vi "SDG60ConfBurstSplit.vi"() -> ()   [LabVIEW 2018]
panel:
  in  "Gate Polarity 0: Positive":u16(ring) items=["Positive", "Negative"]
  in  "Burst Delay (1.352 us)":dbl=1.352e-06
  in  "Triggered/Gated: (0:Triggered)":i32(ring) items=["Triggered", "Gated"]
  in  "Trigger Out Mode (0: Off)":u16(ring) items=["Off", "Rise", "Fall"]
  in  "Trigger Source (0: Internal)":i32(ring) items=["Internal", "External", "Manual"]
  in  "Start Phase (0.0 degrees)":dbl min=0.0 max=360.0 format="%#.15g"
  in  "Channel (1:Channel 1)":i32(ring)=1 items=["Channel 1"=1, "Channel 2"=2]
  in  "Enable Burst (T: Enable)":bool=TRUE
  in  "error in (no error)":errorcluster
  out "error out":errorcluster
  in  "VISA resource name":refnum<visa-resource-name>="USB0::0xF4EC::0x1101::SDG6XEBC5R0119::INSTR"
  out "VISA resource name out":refnum<visa-resource-name>
  # "Trigger out ignored when gated \nand/or TrigSrc is Ext"
  # "Res: 0.1degrees"
  # "Range: 1.352us-100s\nLimited by frequency\n6 digits precision"
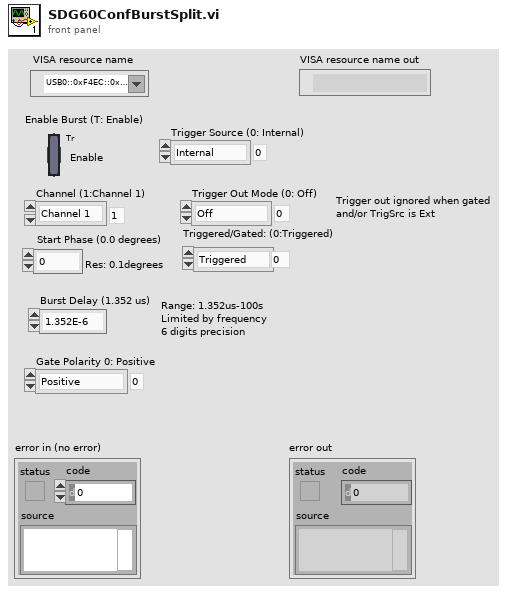
[diagram p1: front panel]
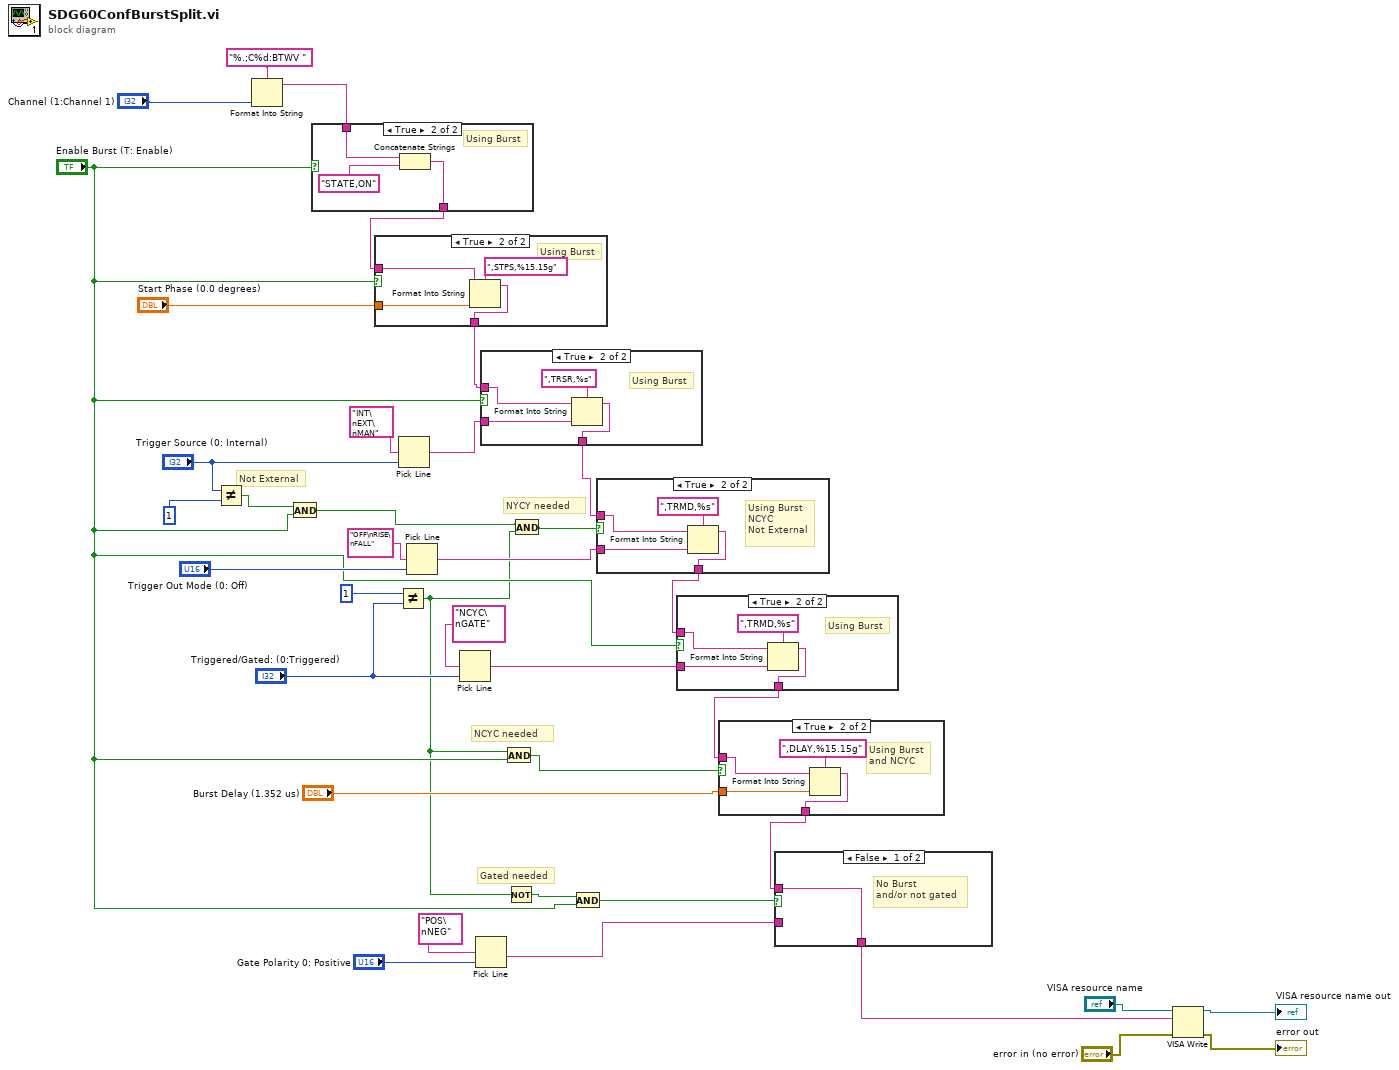
[diagram p0: block diagram]
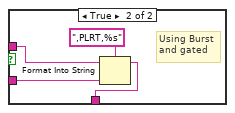
[diagram p2: hidden frame]
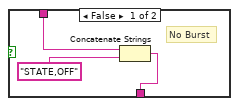
[diagram p8: hidden frame]
diagram:
  # "Gated needed"
  # "NCYC needed"
  # "NYCY needed"
  # "Not External"
  n1 = Not Equal?(x="Trigger Source (0: Internal)", y=1) -> (x != y?=w13:bool)
  n2 = Format Into String(format string="%.;C%d:BTWV ", "Channel (1:Channel 1)") -> (resulting string=w36:string)  [unwired: 2 in, 1 out]
  n3 = And(x=w13, y="Enable Burst (T: Enable)") -> (x .and. y?=w11:bool)
  n4 = case shown="True" "Enable Burst (T: Enable)" {
    tunnel: w36 -> [w41 w44]
    tunnel: [w39 w42] -> w35
    frame False {
      # "No Burst"
      n5 = Concatenate Strings(w41, "STATE,OFF") -> (w39:string)
    }
    frame True {
      # "Using Burst"
      n6 = Concatenate Strings(w44, "STATE,ON") -> (w42:string)
    }
  }
  n7 = case shown="True" "Enable Burst (T: Enable)" {
    tunnel: w35 -> [w45 w48]
    tunnel: [w45 w46] -> w30
    tunnel: "Start Phase (0.0 degrees)" -> [_ w49]
    frame False {
      # "No Burst"
    }
    frame True {
      # "Using Burst"
      n8 = Format Into String(format string=",STPS,%15.15g", initial string=w48, w49) -> (resulting string=w46:string)  [unwired: 1 in, 1 out]
    }
  }
  n9 = Not Equal?(x=1, y="Triggered/Gated: (0:Triggered)") -> (x != y?=w4:bool)
  n10 = Pick Line(multi-line string="INT\nEXT\nMAN", line index="Trigger Source (0: Internal)") -> (output string=w28:string)  [unwired: 1 in]
  n11 = Pick Line(multi-line string="OFF\nRISE\nFALL", line index="Trigger Out Mode (0: Off)") -> (output string=w23:string)  [unwired: 1 in]
  n12 = Pick Line(multi-line string="NCYC\nGATE", line index="Triggered/Gated: (0:Triggered)") -> (output string=w19:string)  [unwired: 1 in]
  n13 = Pick Line(multi-line string="POS\nNEG", line index="Gate Polarity 0: Positive") -> (output string=w2:string)  [unwired: 1 in]
  n14 = case shown="True" "Enable Burst (T: Enable)" {
    tunnel: w30 -> [w50 w54]
    tunnel: [w50 w53] -> w26
    tunnel: w28 -> [_ w52]
    frame False {
      # "No Burst"
    }
    frame True {
      # "Using Burst"
      n15 = Format Into String(format string=",TRSR,%s", initial string=w54, w52) -> (resulting string=w53:string)  [unwired: 1 in, 1 out]
    }
  }
  n16 = And(x=w4, y="Enable Burst (T: Enable)") -> (x .and. y?=w10:bool)
  n17 = Not(x=w4) -> (.not. x?=w7:bool)
  n18 = And(x=w11, y=w4) -> (x .and. y?=w12:bool)
  n19 = And(x=w7, y="Enable Burst (T: Enable)") -> (x .and. y?=w6:bool)
  n20 = case shown="True" w12 {
    tunnel: w26 -> [w55 w59]
    tunnel: [w55 w58] -> w20
    tunnel: w23 -> [_ w57]
    frame False {
      # "not using burst or\ngated or external"
    }
    frame True {
      # "Using Burst\nNCYC\nNot External"
      n21 = Format Into String(format string=",TRMD,%s", initial string=w59, w57) -> (resulting string=w58:string)  [unwired: 1 in, 1 out]
    }
  }
  n22 = case shown="True" "Enable Burst (T: Enable)" {
    tunnel: w20 -> [w60 w64]
    tunnel: [w60 w63] -> w17
    tunnel: w19 -> [_ w61]
    frame False {
      # "No Burst"
    }
    frame True {
      # "Using Burst"
      n23 = Format Into String(format string=",TRMD,%s", initial string=w64, w61) -> (resulting string=w63:string)  [unwired: 1 in, 1 out]
    }
  }
  n24 = case shown="True" w10 {
    tunnel: w17 -> [w65 w69]
    tunnel: "Burst Delay (1.352 us)" -> [_ w67]
    tunnel: [w65 w66] -> w9
    frame False {
      # "No Burst\nand/or gated"
    }
    frame True {
      # "Using Burst\nand NCYC"
      n25 = Format Into String(format string=",DLAY,%15.15g", initial string=w69, w67) -> (resulting string=w66:string)  [unwired: 1 in, 1 out]
    }
  }
  n26 = case shown="False" w6 {
    tunnel: w9 -> [w70 w74]
    tunnel: w2 -> [_ w72]
    tunnel: [w70 w71] -> w8
    frame False {
      # "No Burst\nand/or not gated"
    }
    frame True {
      # "Using Burst\nand gated"
      n27 = Format Into String(format string=",PLRT,%s", initial string=w74, w72) -> (resulting string=w71:string)  [unwired: 1 in, 1 out]
    }
  }
  n28 = VISA Write(VISA resource name="VISA resource name", write buffer=w8, error in (no error)="error in (no error)") -> (VISA resource name out=→"VISA resource name out":refnum<visa-resource-name>, error out=→"error out":errorcluster)  [unwired: 1 out]
